vi "Upgrade Socket to SSL.vi"(8 "error in (no error)":errorcluster, 11 "Socket in":refnum<class "Socket.lvclass">) -> (0 "error out":errorcluster, 3 "dotNET SSL Socket out":refnum<class "dotNET SSL Server.lvclass">)   [LabVIEW 2013, in "dotNET SSL Socket.lvlib" / "dotNET SSL Server.lvclass"]
uses:
  dotNET SSL Server.lvclass
  <vilib>/MediaMongrels Ltd/WebSockets/Sockets/Socket/Socket.lvclass
  dotNET TCP Socket/dotNET TCP Socket.lvclass
  dotNET TCP Socket/dotNET TCP Socket.lvclass/dotNET TCP Socket.ctl
  dotNET SSL Socket/dotNET SSL Socket.lvclass/dotNET SSL Socket.ctl
  dotNET TCP Socket/Read TcpClient.vi
  dotNET SSL Socket/Write SSLStream.vi
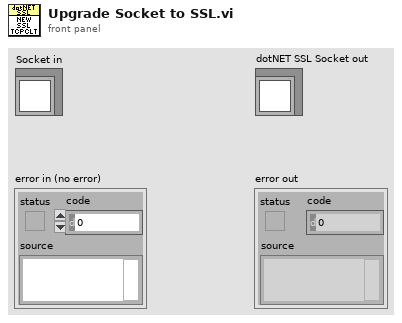
[diagram p1: front panel]
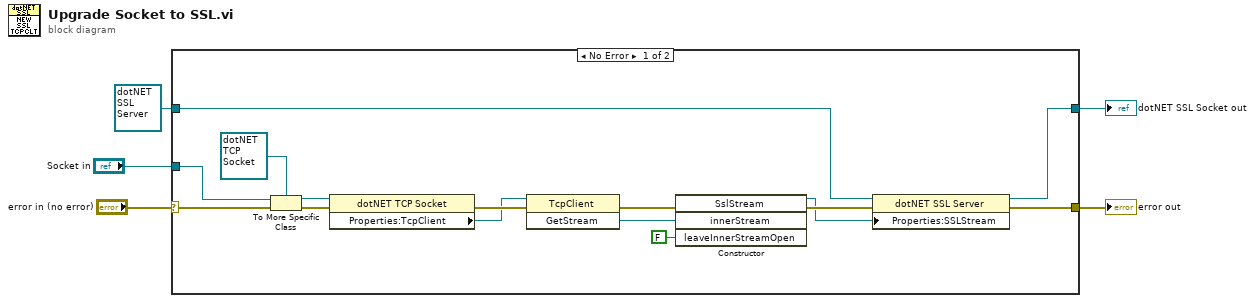
[diagram p0: block diagram]
diagram:
  n1 = case shown="No Error" "error in (no error)" {
    selector: "error in (no error)" -> [w16 w22]
    tunnel: [w14 w22] -> w4
    tunnel: [w12 w21] -> w2
    tunnel: refnum<class "dotNET SSL Server.lvclass"> refnum ("dotNET SSL Socket in") -> [w13 w21]
    tunnel: "Socket in" -> [w10 _]
    frame No Error {
      n2 = To More Specific Class(target class=refnum<class "dotNET TCP Socket.lvclass"> refnum ("dotNET SSL Socket.lvlib:dotNET TCP Socket.lvclass"), reference=w10, error in=w16) -> (specific class reference=w7:refnum<class "dotNET TCP Socket.lvclass">, error out=w11:errorcluster)
      n3 = property class="dotNET TCP Socket"(reference=w7, error in=w11) -> (error out=w8:errorcluster, "Properties:TcpClient"=w6:refnum<k24>)  [unwired: 1 out]
      n4 = invoke class="TcpClient" method="GetStream"(reference=w6, error in=w8) -> (error out=w18:errorcluster, "GetStream"=w20:refnum<k24>)  [unwired: 1 in, 1 out]
      n5 = constructor class="SslStream"(error in=w18, "innerStream"=w20, "leaveInnerStreamOpen"=FALSE) -> (reference out=w15:refnum<k24>, error out=w17:errorcluster)  [unwired: 2 in, 3 out]
      n6 = property class="dotNET SSL Server"(reference=w13, error in=w17, "Properties:SSLStream"=w15) -> (reference out=w12:refnum<class "dotNET SSL Server.lvclass">, error out=w14:errorcluster)
    }
    frame Error {
    }
  }
  "error out" <- w4
  "dotNET SSL Socket out" <- w2
